vi "Checkers Start Screen.vi"   [LabVIEW 2016]
panel:
  # "CHECKERS LAB DEMO"
  # "(Click anywhere to start)"
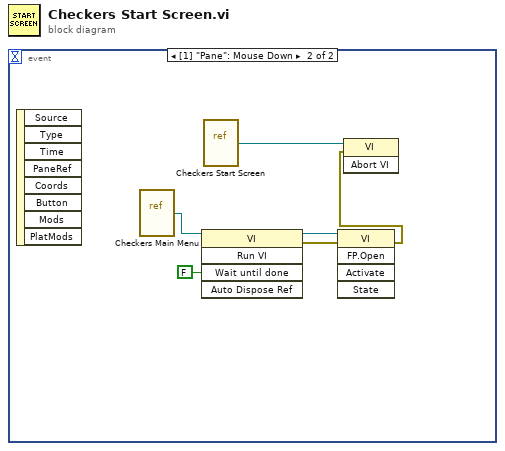
[diagram p0: block diagram]
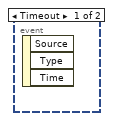
[diagram p2: hidden frame]
diagram:
  n1 = event shown="[1] \"Pane\": Mouse Down" {
    selector: _ -> [_ _]
    dyn-events: _ -> [_ _]
    timeout: _ -> [_ _]
    event Timeout {
      n2 = event-data() -> ()  [unwired: 1 in, 3 out]
    }
    event Mouse Down {
      n3 = event-data() -> ()  [unwired: 1 in, 8 out]
      n4 = vi-ref "Checkers Main Menu.vi"() -> (w6:refnum<vi>)
      n5 = invoke class="VI" method="Run VI"(reference=w6, "Wait until done"=FALSE ("Wait Until Done")) -> (reference out=w5:refnum<vi>, error out=w4:errorcluster)  [unwired: 3 in, 3 out]
      n6 = vi-ref "Checkers Start Screen.vi"() -> (w2:refnum<vi>)
      n7 = invoke class="VI" method="FP.Open"(reference=w5, error in=w4) -> (error out=w3:errorcluster)  [unwired: 3 in, 4 out]
      n8 = invoke class="VI" method="Abort VI"(reference=w2, error in=w3) -> ()  [unwired: 1 in, 3 out]
    }
  }
